vi "getStatus.vi"(0 "Pmx4exSaController in":refnum<class "Pmx4exSaController.lvclass">, 2 "axis (nc - MST commands for the PMX retrieve ALL axes":T5, 5 "error in (no error)":errorcluster) -> (14 "Pmx4exSaController out":refnum<class "Pmx4exSaController.lvclass">, 16 "status (raw result)":string, 17 "full_state":T1={"X"={"motion_state"=enum."CONST", "other_states"=[]}, "Y"={"motion_state"=enum."CONST", "other_states"=[]}, "Z"={"motion_state"=enum."CONST", "other_states"=[]}, "U"={"motion_state"=enum."CONST", "other_states"=[]}, "buffer_enabled?"=FALSE, "buffer_start"=0, "buffer_end"=0, "avail_buffer"=0, "move_mode"=enum."ABSOLUTE"}, 19 "error out":errorcluster)   [LabVIEW 2020, in "classes.lvlib" / "Pmx4exSaController.lvclass"]
doc: "Produced By:\n\n<B>Kod Integrations, LLC</B>\n4835 Marianne Drive\nMount Airy, MD 21771\nhttp://www.kodintegrations.com\nemail: info@kodintegrations.com\nphone: (240) 687-1288"
uses:
  Pmx4exSaController.lvclass
  _Controller.lvclass
  motor_status.ctl
  common.lvlib
  single_axis_state.ctl
  move_mode.ctl
  complete_motor_state.ctl
  C:/GEECS/Developers Version/source/Device Drivers/Newmark-NSC-A/Arcus Driver 3.0.0/ArcusUsbComm/classes/MultiAxisController/_MultiAxisController.lvclass
  C:/GEECS/Developers Version/source/Device Drivers/Newmark-NSC-A/Arcus Driver 3.0.0/ArcusUsbComm/classes/Controller/_Controller.lvclass
  C:/GEECS/Developers Version/source/Device Drivers/Newmark-NSC-A/Arcus Driver 3.0.0/ArcusUsbComm/classes/PMX-4EX-SA/Pmx4exSaController.lvclass
  axis.ctl
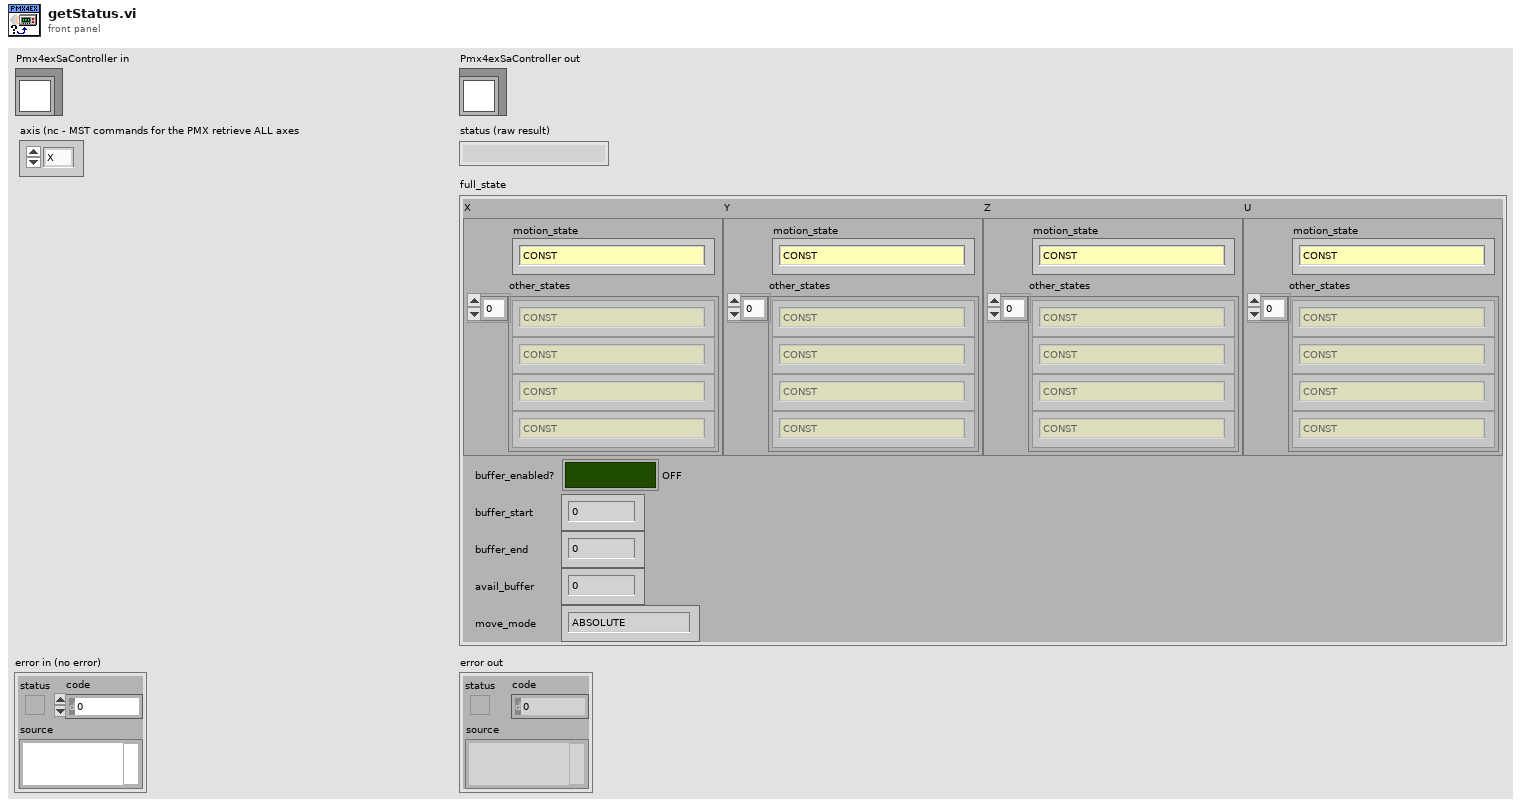
[diagram p1: front panel]
types:
  T1 = typedef "common.lvlib/complete_motor_state.ctl" = cluster{"X":T2, "Y":T2, "Z":T2, "U":T2, "buffer_enabled?":bool, "buffer_start":i32, "buffer_end":i32, "avail_buffer":i32, "move_mode":T4}
  T2 = typedef "common.lvlib/single_axis_state.ctl" = cluster{"motion_state":T3, "other_states":T3[]}
  T3 = typedef "common.lvlib/motor_status.ctl" = enum16{"IDLE", "CONST", "ACCEL", "DECEL", "HOME_SWITCH", "-LIMIT_SWITCH", "+LIMIT_SWITCH", "-LIMIT_ERR", "+LIMIT_ERR", "COMM_TIMEOUT", "ALARM_INPUT", "ALARM_ERROR", "TOC_TIMEOUT_STATUS", "LATCH_INPUT_STATUS", "Z_INDEX_STATUS"}
  T4 = typedef "common.lvlib/move_mode.ctl" = enum16{"ABSOLUTE", "INCREMENTAL"}
  T5 = typedef "common.lvlib/axis.ctl" = enum16{"X", "Y", "Z", "U"}
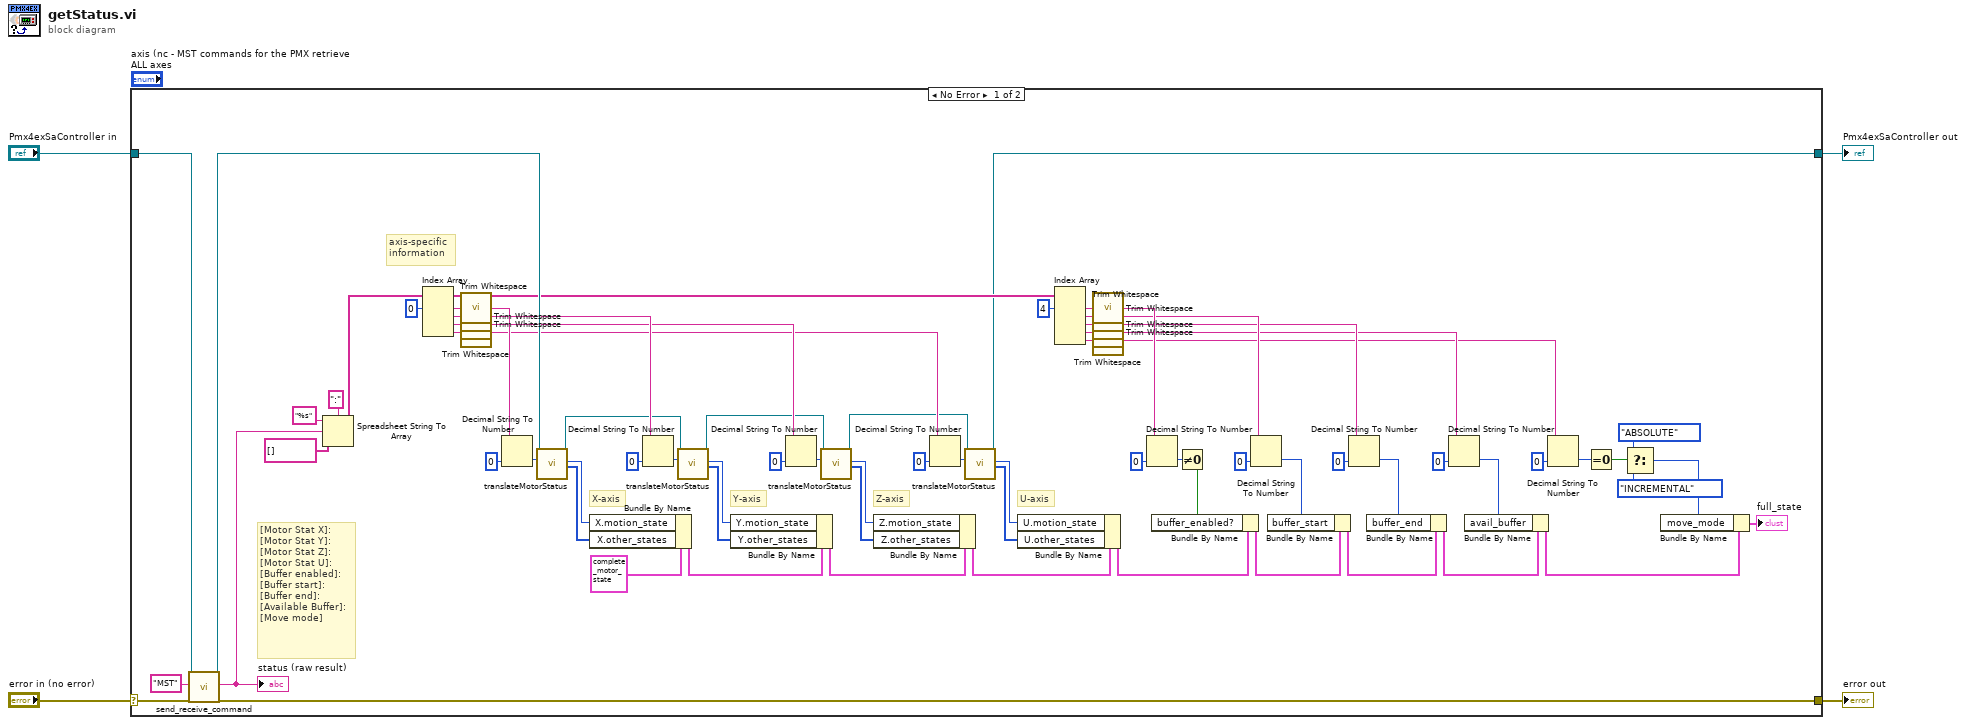
[diagram p0: block diagram]
diagram:
  n1 = case shown="No Error" "error in (no error)" {
    selector: "error in (no error)" -> [w77 w81]
    tunnel: [w76 w81] -> w3
    tunnel: [w31 w80] -> w1
    tunnel: "Pmx4exSaController in" -> [w74 w80]
    frame No Error {
      # "U-axis"
      # "Z-axis"
      # "Y-axis"
      # "X-axis"
      # "axis-specific\ninformation"
      # "[Motor Stat X]:\n[Motor Stat Y]:\n[Motor Stat Z]:\n[Motor Stat U]:\n[Buffer enabled]:\n[Buffer start]:\n[Buffer end]:\n[Available Buffer]:\n[Move mode]"
      n2 = call "send_receive_command.vi"("reference (in)"=w74, "ASCII Command (in)"="MST", "error in (no error)"=w77) -> ("reference (out)"=w73:refnum<class "Pmx4exSaController.lvclass">, "response (out)"=w71:string, "error out"=w76:errorcluster)  [unwired: 12 in, 2 out]
      "status (raw result)" <- w71
      n3 = Spreadsheet String To Array(delimiter (Tab)=":", format string="%s", spreadsheet string=w71, array type (2D Dbl)=string[] []) -> (array=w36:string[])
      n4 = Index Array(array=w36, index #1=0 ("index")) -> (element #1=w67:string, element #2=w66:string, element #3=w65:string, element #4=w64:string)  [unwired: 3 in]
      n5 = call "Trim Whitespace.vi"("string"=w67) -> ("trimmed string"=w63:string)  [unwired: 1 in]
      n6 = call "Trim Whitespace.vi"("string"=w66) -> ("trimmed string"=w55:string)  [unwired: 1 in]
      n7 = call "Trim Whitespace.vi"("string"=w65) -> ("trimmed string"=w46:string)  [unwired: 1 in]
      n8 = call "Trim Whitespace.vi"("string"=w64) -> ("trimmed string"=w45:string)  [unwired: 1 in]
      n9 = Decimal String To Number(string=w63, default (0L)=u32 0 ("default (0 I32)")) -> (number=w78:u32)  [unwired: 1 in, 1 out]
      n10 = call-dynamic "translateMotorStatus.vi"("Pmx4exSaController in"=w73, "actual value"=w78) -> ("Pmx4exSaController out"=w34:refnum<class "Pmx4exSaController.lvclass">, "motion_state"=w61:T3, "other_states"=w60:T3[])  [unwired: 14 in, 1 out]
      n11 = Bundle By Name(cluster=T1 {"X"={"motion_state"=enum."IDLE", "other_states"=[]}, "Y"={"motion_state"=enum."IDLE", "other_states"=[]}, "Z"={"motion_state"=enum."IDLE", "other_states"=[]}, "U"={"motion_state"=enum."IDLE", "other_states"=[]}, "buffer_enabled?"=FALSE, "buffer_start"=0, "buffer_end"=0, "avail_buffer"=0, "move_mode"=enum."INCREMENTAL"} ("full_state"), "X.motion_state"=w61, "X.other_states"=w60) -> (w44:T1)
      n12 = Decimal String To Number(string=w55, default (0L)=u32 0 ("default (0 I32)")) -> (number=w57:u32)  [unwired: 1 in, 1 out]
      n13 = call-dynamic "translateMotorStatus.vi"("Pmx4exSaController in"=w34, "actual value"=w57) -> ("Pmx4exSaController out"=w33:refnum<class "Pmx4exSaController.lvclass">, "motion_state"=w58:T3, "other_states"=w59:T3[])  [unwired: 14 in, 1 out]
      n14 = Bundle By Name(cluster=w44, "Y.motion_state"=w58, "Y.other_states"=w59) -> (w43:T1)
      n15 = Decimal String To Number(string=w46, default (0L)=u32 0 ("default (0 I32)")) -> (number=w53:u32)  [unwired: 1 in, 1 out]
      n16 = call-dynamic "translateMotorStatus.vi"("Pmx4exSaController in"=w33, "actual value"=w53) -> ("Pmx4exSaController out"=w32:refnum<class "Pmx4exSaController.lvclass">, "motion_state"=w52:T3, "other_states"=w51:T3[])  [unwired: 14 in, 1 out]
      n17 = Bundle By Name(cluster=w43, "Z.motion_state"=w52, "Z.other_states"=w51) -> (w42:T1)
      n18 = Decimal String To Number(string=w45, default (0L)=u32 0 ("default (0 I32)")) -> (number=w48:u32)  [unwired: 1 in, 1 out]
      n19 = call-dynamic "translateMotorStatus.vi"("Pmx4exSaController in"=w32, "actual value"=w48) -> ("Pmx4exSaController out"=w31:refnum<class "Pmx4exSaController.lvclass">, "motion_state"=w49:T3, "other_states"=w50:T3[])  [unwired: 14 in, 1 out]
      n20 = Bundle By Name(cluster=w42, "U.motion_state"=w49, "U.other_states"=w50) -> (w26:T1)
      n21 = Index Array(array=w36, index #1=4 ("index")) -> (element #1=w38:string, element #2=w39:string, element #3=w40:string, element #4=w41:string, element #5=w35:string)  [unwired: 4 in]
      n22 = call "Trim Whitespace.vi"("string"=w38) -> ("trimmed string"=w29:string)  [unwired: 1 in]
      n23 = call "Trim Whitespace.vi"("string"=w39) -> ("trimmed string"=w24:string)  [unwired: 1 in]
      n24 = call "Trim Whitespace.vi"("string"=w40) -> ("trimmed string"=w18:string)  [unwired: 1 in]
      n25 = call "Trim Whitespace.vi"("string"=w41) -> ("trimmed string"=w16:string)  [unwired: 1 in]
      n26 = call "Trim Whitespace.vi"("string"=w35) -> ("trimmed string"=w12:string)  [unwired: 1 in]
      n27 = Decimal String To Number(string=w29, default (0L)=u32 0 ("default (0 I32)")) -> (number=w28:u32)  [unwired: 1 in, 1 out]
      n28 = Not Equal To 0?(x=w28) -> (x != 0?=w27:bool)
      n29 = Bundle By Name(cluster=w26, "buffer_enabled?"=w27) -> (w22:T1)
      n30 = Decimal String To Number(string=w24, default (0L)=u32 0 ("default (0 I32)")) -> (number=w23:u32)  [unwired: 1 in, 1 out]
      n31 = Bundle By Name(cluster=w22, "buffer_start"=w23) -> (w19:T1)
      n32 = Decimal String To Number(string=w18, default (0L)=u32 0 ("default (0 I32)")) -> (number=w20:u32)  [unwired: 1 in, 1 out]
      n33 = Bundle By Name(cluster=w19, "buffer_end"=w20) -> (w14:T1)
      n34 = Decimal String To Number(string=w16, default (0L)=u32 0 ("default (0 I32)")) -> (number=w15:u32)  [unwired: 1 in, 1 out]
      n35 = Bundle By Name(cluster=w14, "avail_buffer"=w15) -> (w11:T1)
      n36 = Decimal String To Number(string=w12, default (0L)=u32 0 ("default (0 I32)")) -> (number=w10:u32)  [unwired: 1 in, 1 out]
      n37 = Equal To 0?(x=w10) -> (x = 0?=w9:bool)
      n38 = Select(t=move_mode."ABSOLUTE" ("mode"), s=w9, f=move_mode."INCREMENTAL" ("mode")) -> (s? t:f=w6:T4)
      n39 = Bundle By Name(cluster=w11, "move_mode"=w6) -> (→"full_state":T1)
    }
    frame Error {
    }
  }
  "error out" <- w3
  "Pmx4exSaController out" <- w1
